vi "TCP-Prepend String Length.vi"(4 "Command":string) -> (1 "String":string)   [LabVIEW 2020]
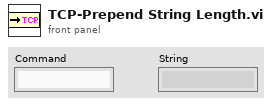
[diagram p1: front panel]
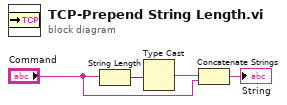
[diagram p0: block diagram]
diagram:
  n1 = String Length(string="Command") -> (length=w1:i32)
  n2 = Type Cast(x=w1) -> (*(type *) &x=w2:string)  [unwired: 1 in]
  n3 = Concatenate Strings(w2, "Command") -> (→"String":string)
